vi "BasicHostWithIFw.vi"() -> ()   [LabVIEW 2017]
uses:
  <instrlib>/_niInstr/FIFO Register Bus/v1/Host/niInstr FIFO Register Bus v1 Host.lvclass
  C:/Program Files (x86)/National Instruments/LabVIEW 2017/instr.lib/_niInstr/Instruction Framework/v1/Host/Instruction Target/niInstr Instruction Target v1 Host.lvclass
  <vilib>/FPGAPlugInAG/sbRIO-9607/niLvFpga_Open_sbRIO-9607.vi
  <vilib>/rvi/interface/common/dynamic/niFpgaDynamicAddResources.vi
  <vilib>/Utility/error.llb/Error Cluster From Error Code.vi
  <vilib>/rvi/errors/niLvFpgaAdjustHostInterfaceError.vi
  <vilib>/FPGAPlugInAG/Dynamic/niLvFpga_Close_Dynamic.vi
  <vilib>/rvi/interface/nirviOpenFPGA/nirviOpenFPGA.xnode
  FPGA Bitfiles/SVPWMdev_FPGATarget_BasicTestWithIFw_aftQj6QlLfU.lvbitx
  <vilib>/rvi/interface/nirviReadWriteControl/nirviReadWriteControl.xnode
  <vilib>/rvi/interface/nirviCloseFPGA/nirviCloseFPGA.xnode
  SVPWMInterface/SVPWMInterface.lvlib
  <instrlib>/_niInstr/Instruction Framework/v1/Host/Subsystem Map/niInstr Subsystem Map v1 Host.lvclass
  NiFpgaLv.dll
  <vilib>/rvi/interface/Simulation/niFpgaSimulationCallBeginRW.vi
panel:
  in  "stop":bool
  out "error out":errorcluster
  out "Period":u32
  out "Deadtime":u8
  in  "modulation":fxp<+/-,16,2>
  in  "freq":sgl
  in  "engauge":bool
  in  "enable":bool
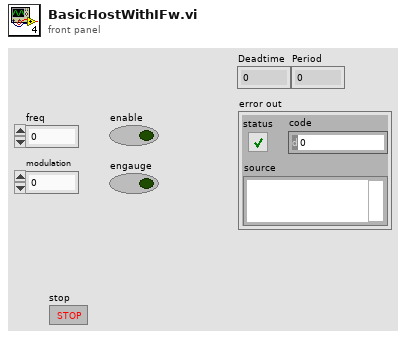
[diagram p1: front panel]
types:
  T1 = typedef "SVPWMInterface.lvlib/Configuration.ctl" = cluster{"Deadtime":u8, "Period":u32}
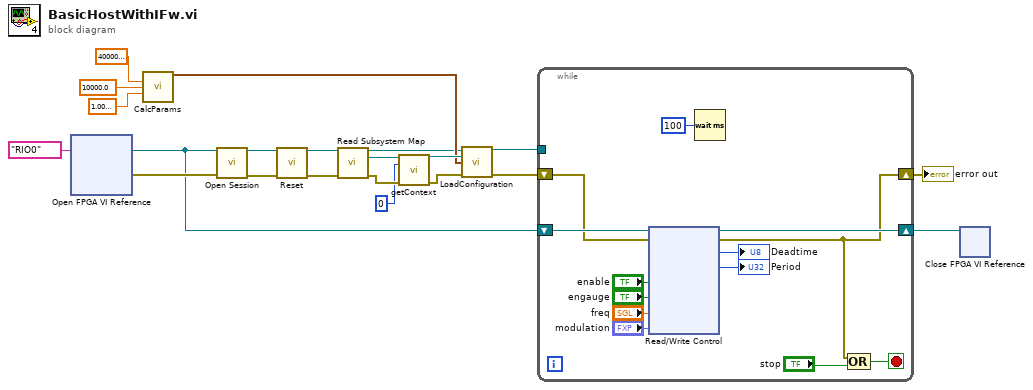
[diagram p0: block diagram]
diagram:
  n1 = xnode "Open FPGA VI Reference"("resource name"=tag "RIO0") -> ("FPGA VI Reference Out"=w6:refnum<k20>, "error out"=w14:errorcluster)  [unwired: 1 in]
  n2 = call "CalcParams.vi"("ClkRate"=sgl 40000000.0, "fc"=sgl 10000.0, "deadtime"=sgl 1e-07) -> ("Configuration"=w9:T1)  [unwired: 12 in]
  n3 = call <instrlib>:"Open Session.vi"("fpga ref"=w6, "error in"=w14) -> ("session out"=w17:refnum<class "niInstr FIFO Register Bus v1 Host.lvclass">, "error out"=w18:errorcluster)  [unwired: 12 in]
  n4 = call-dynamic "Reset.vi"("session in"=w17, "error in"=w18) -> ("session out"=w2:refnum<class "niInstr FIFO Register Bus v1 Host.lvclass">, "error out"=w16:errorcluster)  [unwired: 12 in]
  n5 = call <instrlib>:"Read Subsystem Map.vi"("instruction target in"=w2, "error in"=w16) -> ("instruction target out"=w1:refnum<class "niInstr FIFO Register Bus v1 Host.lvclass">, "subsystem map"=w15:refnum<class "niInstr Subsystem Map v1 Host.lvclass">, "error out"=w13:errorcluster)  [unwired: 11 in]
  n6 = call "getContext.vi"("subsystemMap"=w15, "instance"=u8 0, "error in"=w13) -> ("SVPWMContext"=w11:refnum<class "niInstr Instruction Framework Context v1 Host.lvclass">, "error out"=w12:errorcluster)  [unwired: 11 in]
  n7 = call "LoadConfiguration.vi"("instruction target in"=w1, "SVPWMContext in"=w11, "Configuration"=w9, "error in (no error)"=w12) -> ("instruction target out"=w8:refnum<class "niInstr FIFO Register Bus v1 Host.lvclass">, "error out"=w7:errorcluster)  [unwired: 9 in, 1 out]
  n8 = while {
    tunnel: w8 -> [_]
    shift-right: [w23] -> w4
    shift-left: w7 -> [w33]
    shift-right: [w26] -> w5
    shift-left: w6 -> [w34]
    stop <- w22 stop-if-true
    n9 = xnode "Read/Write Control"("FPGA VI Reference In"=w34, "error in"=w33, "enable"="enable", "engauge"="engauge", "freq"="freq", "modulation"="modulation") -> ("FPGA VI Reference Out"=w26:refnum<k20>, "error out"=w23:errorcluster, "Deadtime"=→"Deadtime":u8, "Period"=→"Period":u32)
    n10 = Wait (ms)(milliseconds to wait=u32 100) -> ()  [unwired: 1 out]
    n11 = Compound Arithmetic op=OR(w23, "stop") -> (w22:bool)
  }
  "error out" <- w4
  n12 = xnode "Close FPGA VI Reference"("FPGA VI Reference In"=w5) -> ()  [unwired: 1 in, 1 out]
